vi "01 - Calling NET.vi"() -> ()   [LabVIEW 2025]
uses:
  C:/Program Files/dotnet/shared/Microsoft.NETCore.App/8.0.20/System.IO.FileSystem.Watcher.dll
  Program Files/dotnet/shared/Microsoft.NETCore.App/8.0.20/System.IO.FileSystem.Watcher.dll
  <vilib>/JDP Science/JSONtext/JSONtext.lvlib
panel:
  in  "Delete":bool
  out "error out":errorcluster
  in  "Overwrite":bool
  out "Last Event":T1
  in  "Stop":bool
  in  "Makefile":bool
  out "Log":string[](array[string]) caption="Log (newest first)"
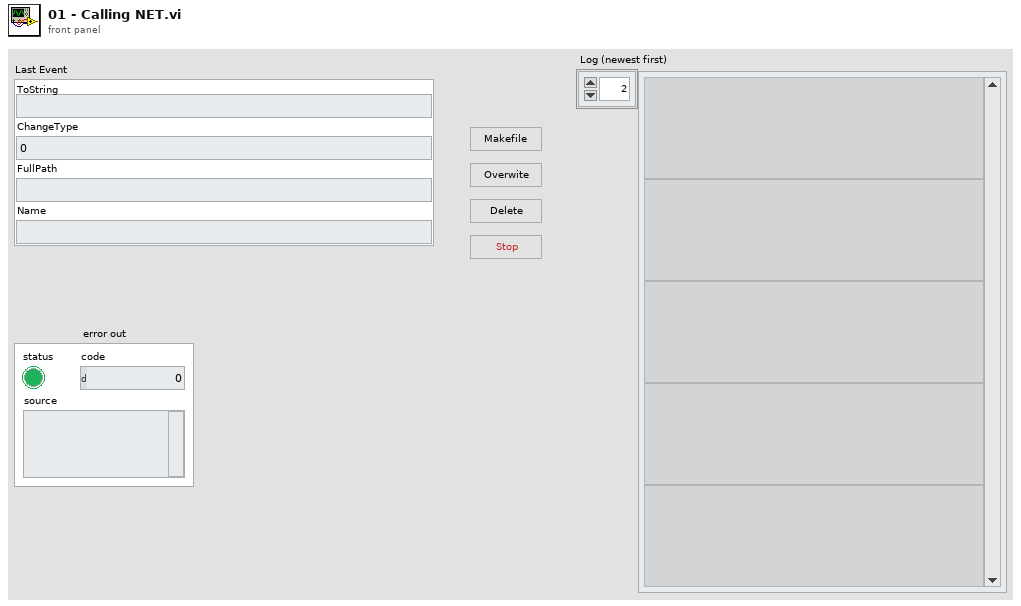
[diagram p1: front panel]
types:
  T1 = cluster{"ToString":string, "ChangeType":dbl, "FullPath":string, "Name":string}
  T2 = cluster{"queue out":refnum<queue>, "notifier out":refnum<notifier>}
  T3 = enum16{"open", "replace", "create", "open or create", "replace or create", "replace or create with confirmation"}
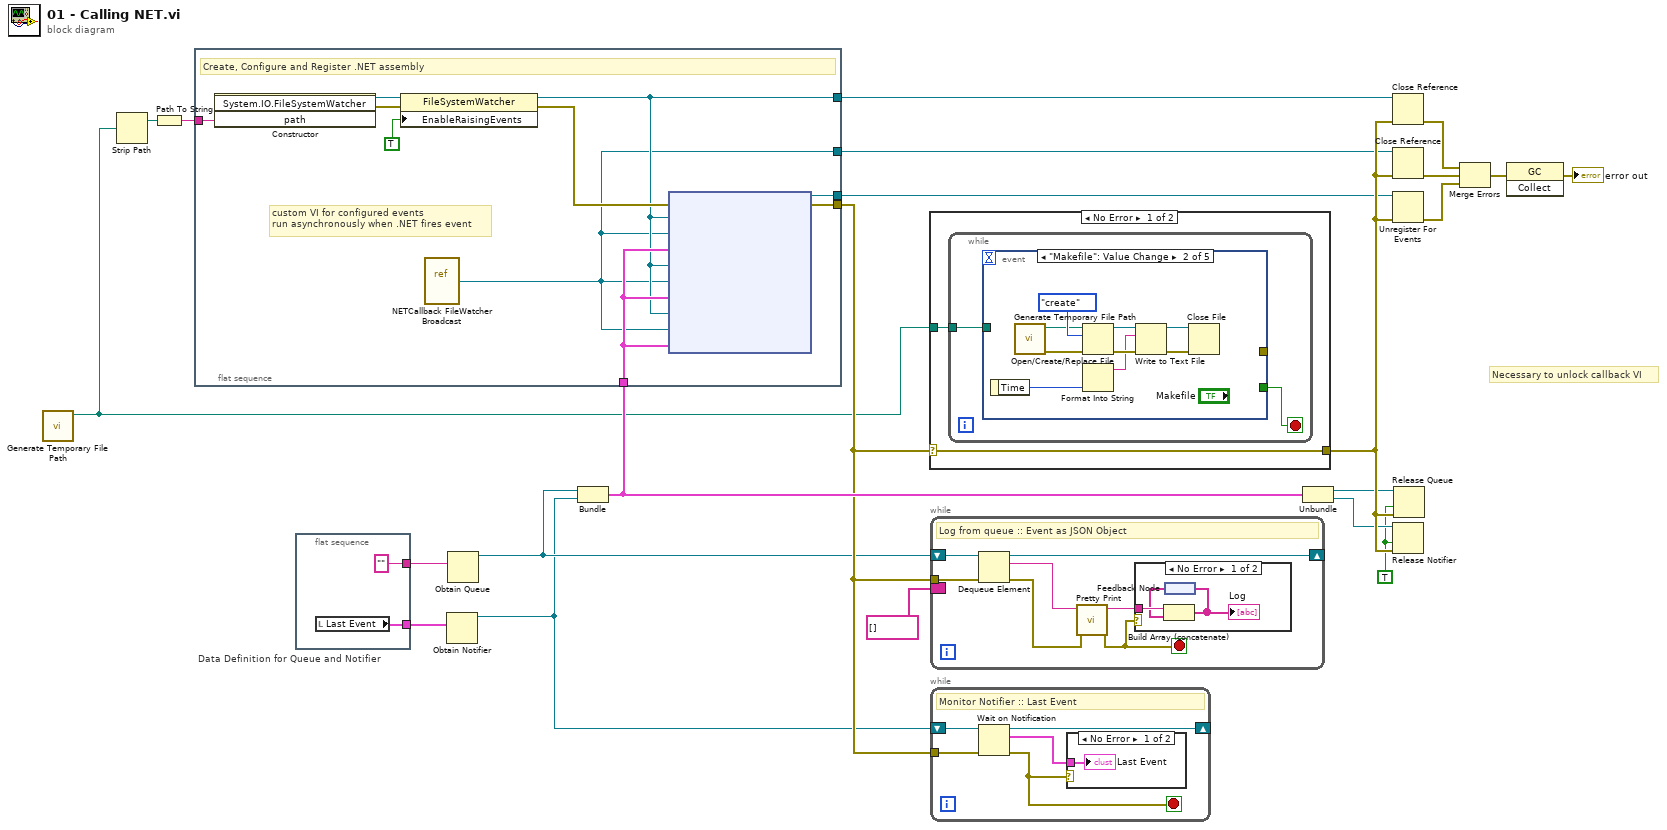
[diagram p0: block diagram]
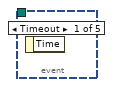
[diagram p2: hidden frame]
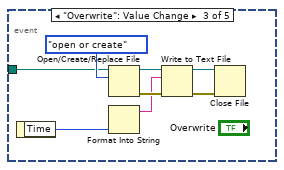
[diagram p3: hidden frame]
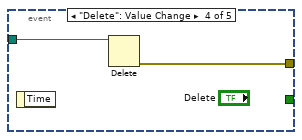
[diagram p4: hidden frame]
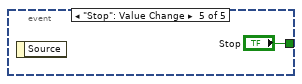
[diagram p5: hidden frame]
diagram:
  w1 = TRUE ("force destroy? (F)")
  # "Necessary to unlock callback VI"
  n1 = call <vilib>:"Generate Temporary File Path.vi"() -> ("Unique Temporary File Path"=w7:path)  [unwired: 10 in, 1 out]
  n2 = Strip Path(path=w7) -> (stripped path=w19:path)  [unwired: 1 out]
  n3 = Path To String(path=w19) -> (string=w18:string)
  n4 = flat-sequence {
    tunnel: w21 -> [w32]
    tunnel: [w31] -> w20
    tunnel: w18 -> [w29]
    tunnel: [w26] -> w13
    tunnel: [w23] -> w9
    tunnel: [w24] -> w4
    frame #0 {
      # "custom VI for configured events\nrun asynchronously when .NET fires event"
      # "Create, Configure and Register .NET assembly"
      n5 = constructor class="FileSystemWatcher"("path"=w29) -> (reference out=w28:refnum<k39>, error out=w27:errorcluster)  [unwired: 3 in, 2 out]
      n6 = property class="FileSystemWatcher"(reference=w28, error in=w27, "EnableRaisingEvents"=TRUE) -> (reference out=w26:refnum<k39>, error out=w30:errorcluster)
      n7 = vi-ref "NETCallback FileWatcher Broadcast.vi"() -> (w23:refnum<vi>)
      n8 = node(w30, w26, w23, w32, w26, w23, w32, w26, w23, w32) -> (w24:refnum<k27>, w31:errorcluster)  [unwired: 1 in]
    }
  }
  n9 = flat-sequence "Data Definition for Queue and Notifier" {
    tunnel: [w34] -> w15
    tunnel: ["" ("name (unnamed)")] -> w14
    frame #0 {
      n10 = local read "Last Event"() -> (w34:T1)
    }
  }
  n11 = Obtain Notifier(notification data type=w15) -> (notifier out=w16:refnum<notifier>)  [unwired: 3 in, 2 out]
  n12 = Obtain Queue(element data type=w14) -> (queue out=w17:refnum<queue>)  [unwired: 4 in, 2 out]
  n13 = Bundle("queue out"=w17, "notifier out"=w16) -> (w21:T2)  [unwired: 1 in]
  n14 = case shown="No Error" w20 {
    selector: w20 -> [w35 w59]
    tunnel: w7 -> [w36 _]
    tunnel: [w35 w59] -> w22
    frame No Error {
      n15 = while {
        tunnel: w36 -> [w38]
        stop <- w37 stop-if-true
        n16 = event shown="[1] \"Makefile\": Value Change" {
          selector: _ -> [_ _ _ _ _]
          dyn-events: _ -> [_ _ _ _ _]
          timeout: _ -> [_ _ _ _ _]
          tunnel: w38 -> [_ _ w48 w57 _]
          tunnel: [_ _ _ _ "Stop"] -> w37
          tunnel: [_ _ _ w56 _] -> _
          event Timeout {
            n17 = event-data() -> ()  [unwired: 1 in, 1 out]
          }
          event "Makefile": Value Change {
            n18 = event-data() -> ("Time"=w42:u32)  [unwired: 1 in]
            n19 = call <vilib>:"Generate Temporary File Path.vi"() -> ("error out"=w39:errorcluster, "Unique Temporary File Path"=w40:path)  [unwired: 10 in]
            n20 = Open/Create/Replace File(file path (use dialog)=w40, error in=w39, operation (0:open)=T3."create") -> (refnum out=w44:refnum<file>, error out=w47:errorcluster)  [unwired: 3 in, 1 out]
            n21 = Format Into String(w42) -> (resulting string=w41:string)  [unwired: 3 in, 1 out]
            n22 = Write to Text File(file (use dialog)=w44, text=w41, error in=w47) -> (refnum out=w43:refnum<file>, error out=w45:errorcluster)  [unwired: 1 in, 1 out]
            n23 = Close File(refnum=w43, error in=w45) -> ()  [unwired: 2 out]
          }
          event "Overwrite": Value Change {
            n24 = event-data() -> ("Time"=w50:u32)  [unwired: 1 in]
            n25 = Open/Create/Replace File(file path (use dialog)=w48, operation (0:open)=T3."open or create") -> (refnum out=w52:refnum<file>, error out=w55:errorcluster)  [unwired: 4 in, 1 out]
            n26 = Format Into String(w50) -> (resulting string=w49:string)  [unwired: 3 in, 1 out]
            n27 = Write to Text File(file (use dialog)=w52, text=w49, error in=w55) -> (refnum out=w51:refnum<file>, error out=w53:errorcluster)  [unwired: 1 in, 1 out]
            n28 = Close File(refnum=w51, error in=w53) -> ()  [unwired: 2 out]
          }
          event "Delete": Value Change {
            n29 = event-data() -> ()  [unwired: 1 in, 1 out]
            n30 = Delete(path (use dialog)=w57) -> (error out=w56:errorcluster)  [unwired: 4 in, 2 out]
          }
          event "Stop": Value Change {
            n31 = event-data() -> ()  [unwired: 1 in, 1 out]
          }
        }
      }
    }
    frame Error {
    }
  }
  n32 = while {
    shift-right: [w65] -> _
    shift-left: w17 -> [w66]
    tunnel: w20 -> [w64]
    border: string[] [] -> [_]
    stop <- w61 stop-if-true
    # "Log from queue :: Event as JSON Object"
    n33 = Dequeue Element(queue=w66, error in (no error)=w64) -> (queue out=w65:refnum<queue>, element=w63:string, error out=w62:errorcluster)  [unwired: 1 in, 1 out]
    n34 = call <vilib>:"Pretty Print.vi"("error in (no error)"=w62, "JSON"=w63) -> ("error out"=w61:errorcluster, "<JSON>"=w60:string)  [unwired: 7 in, 1 out]
    n35 = case shown="No Error" w61 {
      tunnel: w60 -> [w69 _]
      frame No Error {
        n36 = feedback #1() -> (w67:string[])
        n37 = Build Array (concatenate)(w69, w67) -> (w68:string[])
        "Log" <- w68
        n38 = feedback-in #1(w68) -> ()
      }
      frame Error {
      }
    }
  }
  n39 = while {
    shift-right: [w73] -> _
    shift-left: w16 -> [w74]
    tunnel: w20 -> [w72]
    stop <- w70 stop-if-true
    # "Monitor Notifier :: Last Event"
    n40 = Wait on Notification(notifier=w74, error in (no error)=w72) -> (notifier out=w73:refnum<notifier>, notification=w71:T1, error out=w70:errorcluster)  [unwired: 2 in, 1 out]
    n41 = case shown="No Error" w70 {
      tunnel: w71 -> [w75 _]
      frame No Error {
        "Last Event" <- w75
      }
      frame Error {
      }
    }
  }
  n42 = Unbundle(w21) -> ("queue out"=w6:refnum<queue>, "notifier out"=w5:refnum<notifier>)
  n43 = Close Reference(reference=w13, error in (no error)=w22) -> (error out=w10:errorcluster)
  n44 = Close Reference(reference=w9, error in (no error)=w22) -> (error out=w3:errorcluster)
  n45 = Unregister For Events(event registration refnum=w4, error in=w22) -> (error out=w2:errorcluster)
  n46 = Release Notifier(notifier=w5, force destroy? (F)=w1, error in (no error)=w22) -> ()  [unwired: 3 out]
  n47 = Release Queue(queue=w6, force destroy? (F)=w1, error in (no error)=w22) -> ()  [unwired: 3 out]
  n48 = Merge Errors(w10, w3, w2) -> (w11:errorcluster)
  n49 = invoke class="GC" method="Collect"(error in=w11) -> (error out=→"error out":errorcluster)  [unwired: 2 in, 2 out]
